vi "ReadTree.vi"(8 "error in":errorcluster, 10 "root":T1, 11 "repository in":refnum<class "NISE_CEF_HierarchyRepo.lvclass">) -> (0 "error out":errorcluster, 3 "repository out":refnum<class "NISE_CEF_Repository.lvclass">)   [LabVIEW 2013, in "NISE_CEF_HierarchyRepo.lvclass"]
doc: "Transfers information between the repo and the tree control nodes. This should be called before custom views are launched or saving to disk."
uses:
  NISE_CEF_HierarchyRepo.lvclass
  Repository/NISE_CEF_Repository.lvclass
  Node/NodeRef.ctl
  Node/NISE_CEF_Node.lvclass
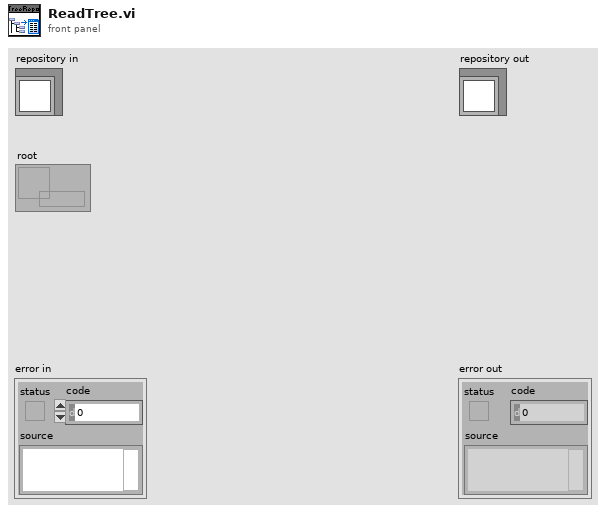
[diagram p1: front panel]
types:
  T1 = typedef "NISE_CEF_Node.lvclass/NodeRef.ctl" = refnum<data-value>
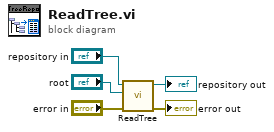
[diagram p0: block diagram]
diagram:
  n1 = call-parent "ReadTree.vi"("error in"="error in", "root"="root", "repository in"="repository in") -> ("error out"=→"error out":errorcluster, "repository out"=→"repository out":refnum<class "NISE_CEF_Repository.lvclass">)  [unwired: 7 in]
